vi "myRIO_BRig_FPGA_v3,0__PortC.vi"() -> ()   [LabVIEW 2014]
uses:
  <vilib>/rvi/FXPMathLib/FxpDiv/subVIs/nifxpmath_Div_SimConfig.ctl
  <vilib>/rvi/FXPMathLib/FxpSinAndCos/subVIs/nifxpmath_SinAndCos_SimConfig.ctl
  <vilib>/rvi/FXPMathLib/FxpDiv/simVIs/DllFxpDivTemp_sub.vi
  <vilib>/rvi/FXPMathLib/FxpSinAndCos/simVIs/DllFxpSinAndCosTemp_sub.vi
  <vilib>/rvi/Emulation/niFpgaGetClockAttributes.vi
  <vilib>/rvi/Emulation/niFpgaSctlEmulationGetInTimedLoop.vi
  <vilib>/rvi/Emulation/niFpgaEmulationReportErrorSimple.vi
  <vilib>/rvi/eio/common/nirviEmuTemplateMethod_errors.vi
  <vilib>/rvi/Emulation/niFpgaCriticalErrorInLSC.vi
  <vilib>/rvi/FXPMathLib/FxpDiv/XNode/nifxpmath_Div.xnode
  <vilib>/rvi/FXPMathLib/FxpMul/XNode/nifxpmath_Multiplier.xnode
  <vilib>/rvi/FXPMathLib/FxpSinAndCos/XNode/nifxpmath_SinAndCos.xnode
  <vilib>/rvi/FXPMathLib/FxpSub/XNode/nifxpmath_Sub.xnode
  <vilib>/eio/EIONode/EIONode.xnode
  <vilib>/rvi/FXPMathLib/sim/FxpSim.dll
panel:
  in  "f_time_select":u32=173
  in  "laser_Nvalley":u32=100
  in  "laser_Npeak":u32=100
  in  "laserledMTrig":bool
  in  "tCycle_laser_wro":u32=100
  in  "tDelay_laser_wro":u32
  in  "tCycle_laser_rew":u32=100
  in  "tDelay_laser_rew":u32
  in  "laserResponse_reward_LED":bool
  in  "laserResponse_wrong_LED":bool
  out "SelectWrong":bool
  out "SelectReward":bool
  in  "laserResponse_wrong":bool
  in  "laserResponse_reward":bool
  in  "Left(F)_or_Right(T)":bool
  in  "ignoreWrong":bool
  in  "SelectionState":bool
  in  "laserMTrig":bool
  in  "FPGA_Stop":bool
  in  "audioTrigger_L":bool
  in  "audioTrigger_R":bool
  in  "audioFreq_L_Hz":u16=1000 min=1000 max=14000 step=1000
  in  "audioAmp_L":u16=1 min=1 max=32767 step=1
  in  "audioFreq_R_Hz":u16=1000 min=1000 max=14000 step=1000
  in  "audioAmp_R":u16=1 min=1 max=32767 step=1
  in  "A3_SL":bool
  in  "A1_SR":bool
  in  "Counts_Reset":bool
  out "A4_LickR":u32
  out "A2_LickL":u32
  in  "A6_Act":bool
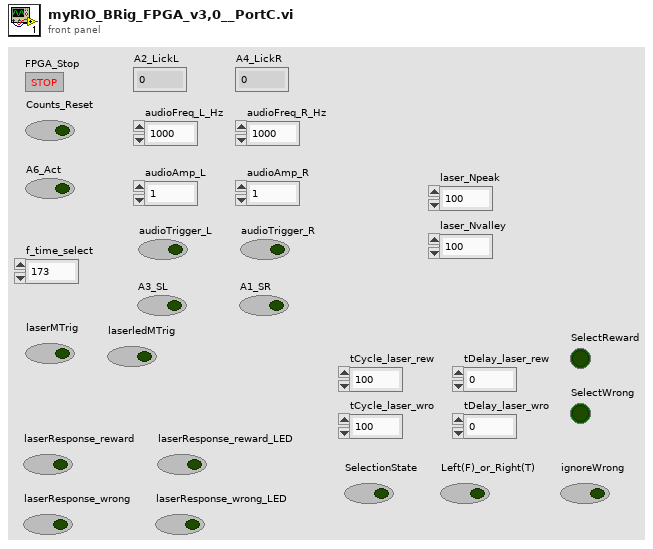
[diagram p1: front panel]
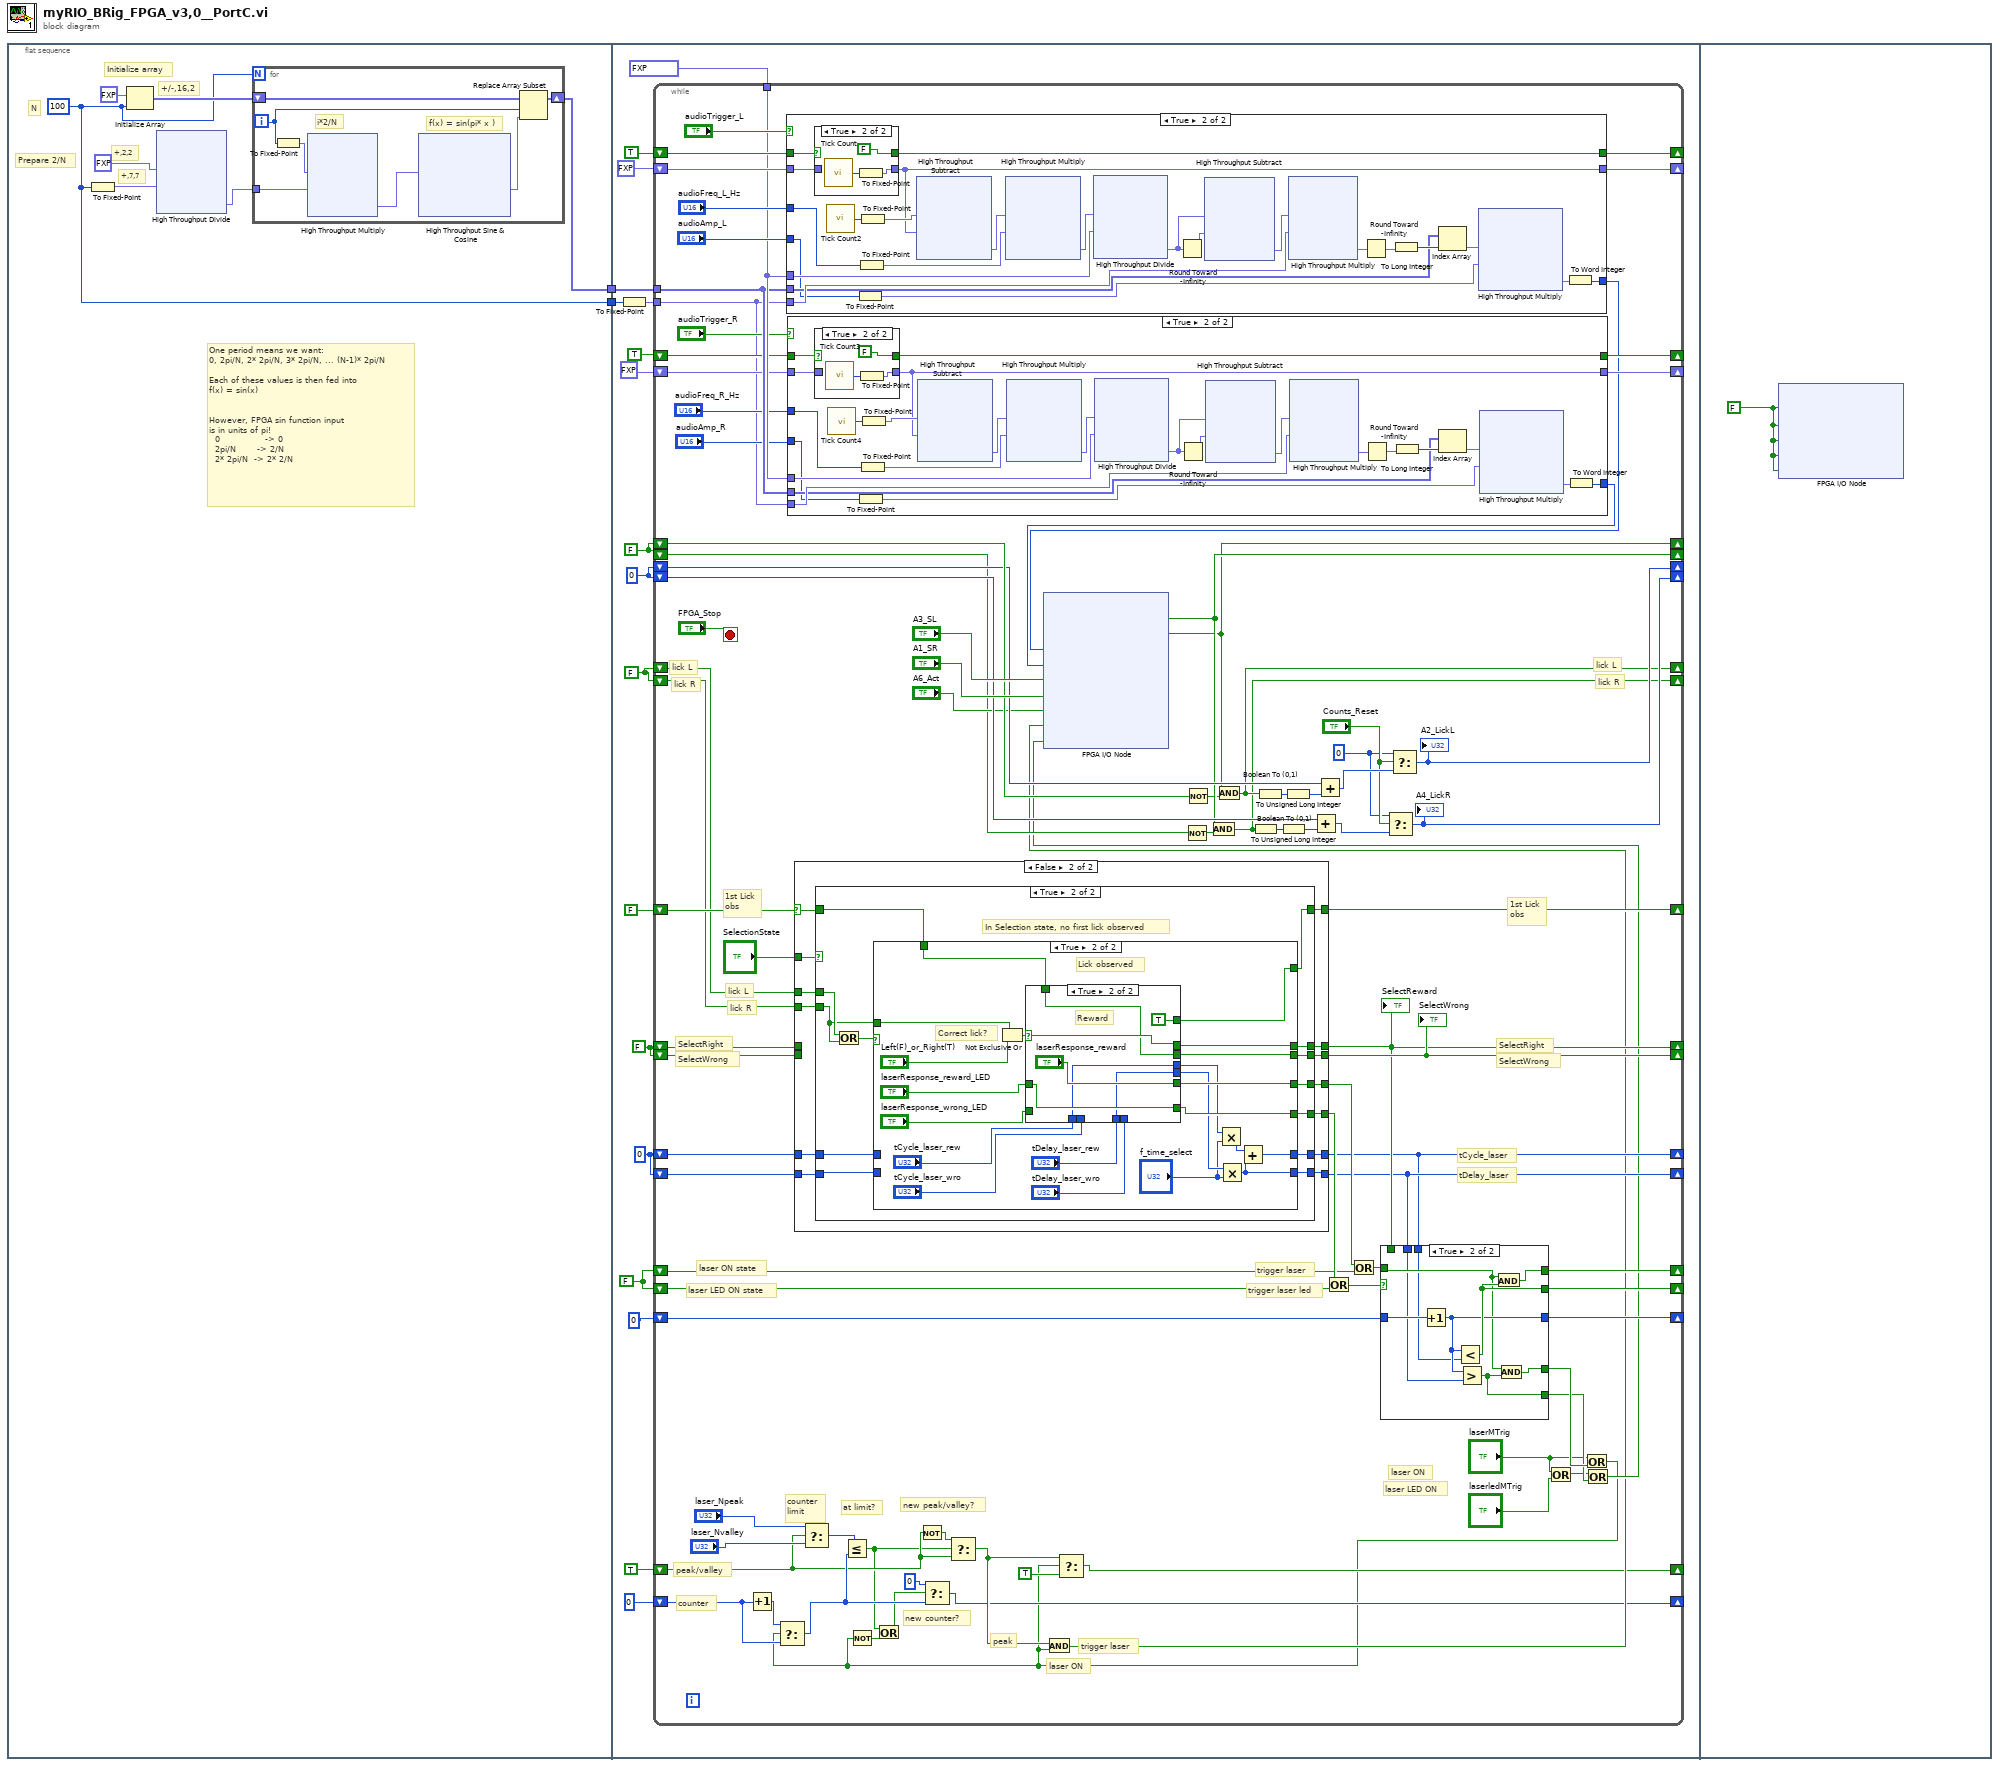
[diagram p0: block diagram]
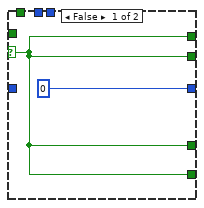
[diagram p2: hidden frame]
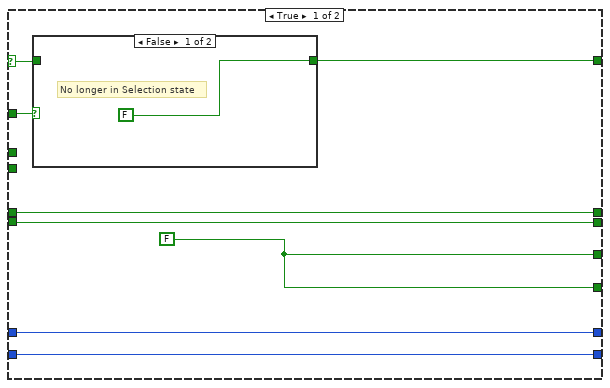
[diagram p3: hidden frame]
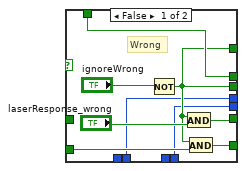
[diagram p7: hidden frame]
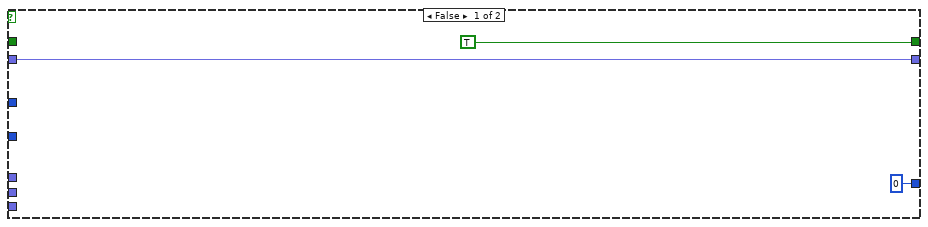
[diagram p8: hidden frame]
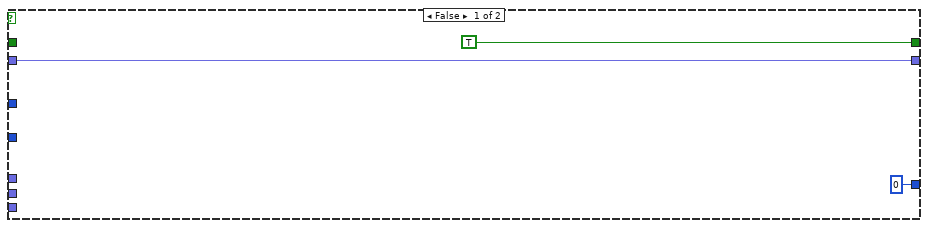
[diagram p10: hidden frame]
diagram:
  n1 = flat-sequence {
    tunnel: [w4] -> w2
    tunnel: [w3] -> w1
    tunnel: w2 -> [w86]
    tunnel: w1 -> [w88]
    frame #0 {
      w3 = 100 ("dimension size")
      # "N"
      # "+,7,7"
      # "+,2,2"
      # "+/-,16,2"
      # "Prepare 2/N"
      # "One period means we want:\n0, 2pi/N, 2* 2pi/N, 3* 2pi/N, ... (N-1)* 2pi/N\n\nEach of these values is then fed into\nf(x) = sin(x)\n\n\nHowever, FPGA sin function input\nis in units of pi!\n  0               -> 0\n  2pi/N       -> 2/N\n  2* 2pi/N  -> 2* 2/N"
      # "Initialize array"
      n2 = To Fixed-Point(number=w3) -> (fixed-point=w6:fxp<+,7,7>)  [unwired: 1 in]
      n3 = Initialize Array(fxp<+/-,16,2> 0.0 ("element"), w3) -> (w9:fxp<+/-,16,2>[])
      n4 = xnode "High Throughput Divide"("x"=fxp<+,2,2> 2.0, "y"=w6) -> ("x/y"=w5:fxp<+,27,0>)
      n5 = for {
        N: w3 -> [_]
        shift-right: [w42] -> w4
        shift-left: w9 -> [w43]
        tunnel: w5 -> [w38]
        i -> [w41]
        # "f(x) = sin(pi* x )"
        # "i*2/N"
        n6 = To Fixed-Point(number=w41) -> (fixed-point=w39:fxp<+,7,7>)  [unwired: 1 in]
        n7 = xnode ("High Throughput Multiply")("x"=w39, "y"=w38) -> ("x*y"=w37:fxp<+,34,7>)
        n8 = xnode "High Throughput Sine & Cosine"("x (pi)"=w37) -> ("sin(x)"=w40:fxp<+/-,16,2>)  [unwired: 1 out]
        n9 = Replace Array Subset(array=w43, new element=w40, index=w41) -> (w42:fxp<+/-,16,2>[])
      }
    }
    frame #1 {
      w76 = u32 0
      w78 = FALSE
      w77 = FALSE
      w81 = FALSE
      w82 = FALSE
      w83 = u32 0
      n10 = To Fixed-Point(number=w88) -> (fixed-point=w87:fxp<+,7,7>)  [unwired: 1 in]
      n11 = while {
        shift-right: [w175] -> _
        shift-left: TRUE -> [w179]
        shift-right: [w174] -> _
        shift-left: fxp<+,32,32> 0.0 -> [w178]
        tunnel: fxp<+,17,26> 40000000.0 -> [w173]
        tunnel: w87 -> [w166]
        tunnel: w86 -> [w172]
        shift-right: [w165] -> _
        shift-left: TRUE -> [w171]
        shift-right: [w164] -> _
        shift-left: fxp<+,32,32> 0.0 -> [w170]
        shift-right: [w141] -> _
        shift-left: w83 -> [w153]
        shift-right: [w144] -> _
        shift-left: w83 -> [w157]
        shift-right: [w145] -> _
        shift-left: w82 -> [w148]
        shift-right: [w142] -> _
        shift-left: w82 -> [w154]
        shift-right: [w139] -> _
        shift-left: FALSE -> [w138]
        shift-right: [w137] -> _
        shift-left: w81 -> [w135]
        shift-right: [w136] -> _
        shift-left: w81 -> [w134]
        shift-right: [w124] -> _
        shift-left: w77 -> [w126]
        shift-right: [w132] -> _
        shift-left: u32 0 -> [w133]
        shift-right: [w118] -> _
        shift-left: w78 -> [w130]
        shift-right: [w131] -> _
        shift-left: w78 -> [w129]
        shift-right: [w125] -> _
        shift-left: w77 -> [w122]
        shift-right: [w114] -> _
        shift-left: w76 -> [w117]
        shift-right: [w115] -> _
        shift-left: w76 -> [w116]
        shift-right: [w96] -> _
        shift-left: u32 0 -> [w108]
        shift-right: [w97] -> _
        shift-left: TRUE -> [w100]
        stop <- "FPGA_Stop" stop-if-true
        w150 = u32 0
        # "trigger laser"
        # "peak"
        # "laser ON"
        # "new peak/valley?"
        # "counter"
        # "peak/valley"
        # "new counter?"
        # "at limit?"
        # "counter\nlimit"
        # "tDelay_laser"
        # "tCycle_laser"
        # "laser LED ON"
        # "laser ON"
        # "laser LED ON state"
        # "laser ON state"
        # "SelectWrong"
        # "SelectRight"
        # "SelectWrong"
        # "SelectRight"
        # "lick R"
        # "lick L"
        # "1st Lick\nobs"
        # "1st Lick\nobs"
        # "lick R"
        # "lick L"
        # "lick R"
        # "lick L"
        # "trigger laser led"
        # "trigger laser"
        n12 = Increment(x=w108) -> (x+1=w106:u32)
        n13 = case shown="True" "audioTrigger_L" {
          tunnel: w179 -> [_ w357]
          tunnel: w178 -> [w333 w356]
          tunnel: "audioFreq_L_Hz" -> [_ w353]
          tunnel: w173 -> [_ w350]
          tunnel: [w333 w334] -> w174
          tunnel: [TRUE w347] -> w175
          tunnel: w166 -> [_ w346]
          tunnel: w172 -> [_ w341]
          tunnel: "audioAmp_L" -> [_ w339]
          tunnel: [i16 0 w336] -> w160
          frame False {
          }
          frame True {
            n14 = case shown="True" w357 {
              selector: w357 -> [w386 _]
              tunnel: [w386 FALSE] -> w347
              tunnel: w356 -> [w385 _]
              tunnel: [w385 w387] -> w334
              frame False {
              }
              frame True {
                n15 = call "Tick Count"() -> ("Tick Count(Ticks)"=w389:u32)
                n16 = To Fixed-Point(number=w389) -> (fixed-point=w387:fxp<+,32,32>)  [unwired: 1 in]
              }
            }
            n17 = call "Tick Count2"() -> ("Tick Count(Ticks)"=w355:u32)
            n18 = To Fixed-Point(number=w339) -> (fixed-point=w338:fxp<+,15,15>)  [unwired: 1 in]
            n19 = To Fixed-Point(number=w353) -> (fixed-point=w352:fxp<+,14,14>)  [unwired: 1 in]
            n20 = To Fixed-Point(number=w355) -> (fixed-point=w335:fxp<+,32,32>)  [unwired: 1 in]
            n21 = xnode "High Throughput Subtract"("x"=w335, "y"=w334) -> ("x-y"=w354:fxp<+,32,32>)
            n22 = xnode ("High Throughput Multiply")("x"=w354, "y"=w352) -> ("x*y"=w351:fxp<+,46,46>)
            n23 = xnode "High Throughput Divide"("x"=w351, "y"=w350) -> ("x/y"=w349:fxp<+,34,21>)
            n24 = Round Toward -Infinity(1:w349) -> (0:w348:fxp<+,21,21>)
            n25 = xnode "High Throughput Subtract"("x"=w349, "y"=w348) -> ("x-y"=w345:fxp<+,14,1>)
            n26 = xnode ("High Throughput Multiply")("x"=w345, "y"=w346) -> ("x*y"=w342:fxp<+,21,8>)
            n27 = Round Toward -Infinity(1:w342) -> (0:w344:fxp<+,8,8>)
            n28 = To Long Integer(number=w344) -> (32bit integer=w343:i32)
            n29 = Index Array(array=w341, index=w343) -> (element=w340:fxp<+/-,16,2>)
            n30 = xnode ("High Throughput Multiply")("x"=w340, "y"=w338) -> ("x*y"=w337:fxp<+/-,31,17>)
            n31 = To Word Integer(number=w337) -> (16bit integer=w336:i16)
          }
        }
        n32 = case shown="True" "audioTrigger_R" {
          tunnel: w171 -> [_ w298]
          tunnel: w170 -> [w274 w297]
          tunnel: "audioFreq_R_Hz" -> [_ w294]
          tunnel: w173 -> [_ w291]
          tunnel: [w274 w275] -> w164
          tunnel: [TRUE w288] -> w165
          tunnel: w166 -> [_ w287]
          tunnel: w172 -> [_ w282]
          tunnel: "audioAmp_R" -> [_ w280]
          tunnel: [i16 0 w277] -> w161
          frame False {
          }
          frame True {
            n33 = case shown="True" w298 {
              selector: w298 -> [w327 _]
              tunnel: [w327 FALSE] -> w288
              tunnel: w297 -> [w326 _]
              tunnel: [w326 w328] -> w275
              frame False {
              }
              frame True {
                n34 = call "Tick Count3"() -> ("Tick Count(Ticks)"=w330:u32)
                n35 = To Fixed-Point(number=w330) -> (fixed-point=w328:fxp<+,32,32>)  [unwired: 1 in]
              }
            }
            n36 = call "Tick Count4"() -> ("Tick Count(Ticks)"=w296:u32)
            n37 = To Fixed-Point(number=w280) -> (fixed-point=w279:fxp<+,15,15>)  [unwired: 1 in]
            n38 = To Fixed-Point(number=w294) -> (fixed-point=w293:fxp<+,14,14>)  [unwired: 1 in]
            n39 = To Fixed-Point(number=w296) -> (fixed-point=w276:fxp<+,32,32>)  [unwired: 1 in]
            n40 = xnode "High Throughput Subtract"("x"=w276, "y"=w275) -> ("x-y"=w295:fxp<+,32,32>)
            n41 = xnode ("High Throughput Multiply")("x"=w295, "y"=w293) -> ("x*y"=w292:fxp<+,46,46>)
            n42 = xnode "High Throughput Divide"("x"=w292, "y"=w291) -> ("x/y"=w290:fxp<+,34,21>)
            n43 = Round Toward -Infinity(1:w290) -> (0:w289:fxp<+,21,21>)
            n44 = xnode "High Throughput Subtract"("x"=w290, "y"=w289) -> ("x-y"=w286:fxp<+,14,1>)
            n45 = xnode ("High Throughput Multiply")("x"=w286, "y"=w287) -> ("x*y"=w283:fxp<+,21,8>)
            n46 = Round Toward -Infinity(1:w283) -> (0:w285:fxp<+,8,8>)
            n47 = To Long Integer(number=w285) -> (32bit integer=w284:i32)
            n48 = Index Array(array=w282, index=w284) -> (element=w281:fxp<+/-,16,2>)
            n49 = xnode ("High Throughput Multiply")("x"=w281, "y"=w279) -> ("x*y"=w278:fxp<+/-,31,17>)
            n50 = To Word Integer(number=w278) -> (16bit integer=w277:i16)
          }
        }
        n51 = case shown="False" w138 {
          selector: w138 -> [w198 w213]
          tunnel: "SelectionState" -> [w200 w215]
          tunnel: [w199 w214] -> w139
          tunnel: w135 -> [_ w212]
          tunnel: w134 -> [_ w211]
          tunnel: [w197 w210] -> w123
          tunnel: [w195 w209] -> w118
          tunnel: [w196 w208] -> w131
          tunnel: w130 -> [w195 _]
          tunnel: w129 -> [w196 _]
          tunnel: [w197 w207] -> w127
          tunnel: [w194 w206] -> w114
          tunnel: [w193 w205] -> w115
          tunnel: w117 -> [w194 w204]
          tunnel: w116 -> [w193 w203]
          frame True {
            w197 = FALSE
            n52 = case shown="False" w200 {
              tunnel: [FALSE w202] -> w199
              tunnel: w198 -> [_ w202]
              frame False {
                # "No longer in Selection state"
              }
              frame True {
                # "Already observed first lick, no other action"
              }
            }
          }
          frame False {
            n53 = case shown="True" w215 {
              tunnel: [w218 w228] -> w214
              tunnel: w213 -> [w218 w224]
              tunnel: w212 -> [_ w230]
              tunnel: w211 -> [_ w229]
              tunnel: [w218 w227] -> w210
              tunnel: [w218 w226] -> w209
              tunnel: [w218 w225] -> w208
              tunnel: [w218 w223] -> w207
              tunnel: [w217 w222] -> w206
              tunnel: [w216 w221] -> w205
              tunnel: w204 -> [w217 w220]
              tunnel: w203 -> [w216 w219]
              frame False {
                # "Not in Selection state"
              }
              frame True {
                # "In Selection state, no first lick observed"
                n54 = Or(x=w230, y=w229) -> (x .or. y?=w231:bool)
                n55 = case shown="True" w231 {
                  tunnel: w229 -> [_ w254]
                  tunnel: [w234 w247] -> w228
                  tunnel: [w234 w252] -> w227
                  tunnel: [w234 w251] -> w226
                  tunnel: [w234 w250] -> w225
                  tunnel: w224 -> [w234 w249]
                  tunnel: [w234 w248] -> w223
                  tunnel: [w233 w236] -> w222
                  tunnel: [w232 w235] -> w221
                  tunnel: w220 -> [w233 _]
                  tunnel: w219 -> [w232 _]
                  frame False {
                  }
                  frame True {
                    # "Correct lick?"
                    # "Lick observed"
                    n56 = Not Exclusive Or(1:"Left(F)_or_Right(T)", 2:w254) -> (0:w253:bool)
                    n57 = case shown="True" w253 {
                      selector: w253 -> [_ w270]
                      tunnel: [w261 "laserResponse_reward"] -> w252
                      tunnel: [w259 w266] -> w250
                      tunnel: [w263 w270] -> w251
                      tunnel: w249 -> [w263 w266]
                      tunnel: [w260 w268] -> w248
                      tunnel: [w259 TRUE] -> w247
                      tunnel: "laserResponse_reward_LED" -> [_ w268]
                      tunnel: "laserResponse_wrong_LED" -> [w258 _]
                      tunnel: "tCycle_laser_rew" -> [_ w265]
                      tunnel: "tCycle_laser_wro" -> [w256 _]
                      tunnel: "tDelay_laser_rew" -> [_ w267]
                      tunnel: "tDelay_laser_wro" -> [w257 _]
                      tunnel: [w257 w267] -> w239
                      tunnel: [w256 w265] -> w238
                      frame False {
                        # "Wrong"
                        n58 = Not(x="ignoreWrong") -> (.not. x?=w259:bool)
                        n59 = And(x=w259, y="laserResponse_wrong") -> (x .and. y?=w261:bool)
                        n60 = And(x=w259, y=w258) -> (x .and. y?=w260:bool)
                      }
                      frame True {
                        # "Reward"
                      }
                    }
                    n61 = Multiply(x=w238, y="f_time_select") -> (x*y=w240:u32)
                    n62 = Multiply(x=w239, y="f_time_select") -> (x*y=w235:u32)
                    n63 = Add(x=w240, y=w235) -> (x+y=w236:u32)
                  }
                }
              }
            }
          }
        }
        "SelectWrong" <- w131
        "SelectReward" <- w118
        n64 = Select(t="laser_Npeak", s=w100, f="laser_Nvalley") -> (s? t:f=w110:u32)
        n65 = Not(x=w100) -> (.not. x?=w101:bool)
        n66 = Not(x=w148) -> (.not. x?=w147:bool)
        n67 = Not(x=w154) -> (.not. x?=w143:bool)
        n68 = Or(x=w127, y=w126) -> (x .or. y?=w128:bool)
        n69 = Or(x=w123, y=w122) -> (x .or. y?=w121:bool)
        n70 = case shown="True" w128 {
          selector: w128 -> [w182 _]
          tunnel: w133 -> [_ w192]
          tunnel: [u32 0 w189] -> w132
          tunnel: [w182 w190] -> w124
          tunnel: [w182 w191] -> w125
          tunnel: w121 -> [_ w188]
          tunnel: [w182 w187] -> w119
          tunnel: [w182 w186] -> w120
          tunnel: w118 -> [_ _]
          tunnel: w115 -> [_ w185]
          tunnel: w114 -> [_ w184]
          frame False {
          }
          frame True {
            n71 = Increment(x=w192) -> (x+1=w189:u32)
            n72 = Less?(x=w189, y=w184) -> (x < y?=w190:bool)
            n73 = Greater?(x=w189, y=w185) -> (0:w187:bool)
            n74 = And(x=w188, y=w190) -> (x .and. y?=w191:bool)
            n75 = And(x=w188, y=w187) -> (x .and. y?=w186:bool)
          }
        }
        n76 = Or(x="laserMTrig", y="laserledMTrig") -> (x .or. y?=w112:bool)
        n77 = Or(x="laserMTrig", y=w120) -> (x .or. y?=w94:bool)
        n78 = Select(t=w106, s=w94, f=w108) -> (s? t:f=w105:u32)
        n79 = Less Or Equal?(x=w110, y=w105) -> (x <= y?=w93:bool)
        n80 = Not(x=w94) -> (.not. x?=w95:bool)
        n81 = Or(x=w93, y=w95) -> (x .or. y?=w92:bool)
        n82 = Select(t=u32 0, s=w92, f=w105) -> (s? t:f=w96:u32)
        n83 = Select(t=w101, s=w93, f=w100) -> (s? t:f=w99:bool)
        n84 = And(x=w99, y=w94) -> (x .and. y?=w102:bool)
        n85 = Select(t=w99, s=w94, f=TRUE) -> (s? t:f=w97:bool)
        n86 = Or(x=w112, y=w119) -> (x .or. y?=w107:bool)
        n87 = xnode "FPGA I/O Node"("AudioOut/Left"=w160, "AudioOut/Right"=w161, "ConnectorC/DIO3"="A3_SL", "ConnectorC/DIO1"="A1_SR", "ConnectorC/DIO6"="A6_Act", "ConnectorC/DIO0"=w102, "ConnectorC/DIO7"=w107) -> ("ConnectorC/DIO4"=w145:bool, "ConnectorC/DIO2"=w142:bool)  [unwired: 9 in, 9 out]
        n88 = And(x=w145, y=w147) -> (x .and. y?=w136:bool)
        n89 = And(x=w142, y=w143) -> (x .and. y?=w137:bool)
        n90 = Boolean To (0,1)(Boolean=w136) -> (0, 1=w159:i16)
        n91 = Boolean To (0,1)(Boolean=w137) -> (0, 1=w156:i16)
        n92 = To Unsigned Long Integer(number=w159) -> (unsigned 32bit integer=w158:u32)
        n93 = To Unsigned Long Integer(number=w156) -> (unsigned 32bit integer=w155:u32)
        n94 = Add(x=w157, y=w158) -> (x+y=w146:u32)
        n95 = Add(x=w153, y=w155) -> (x+y=w152:u32)
        n96 = Select(t=w150, s="Counts_Reset", f=w146) -> (s? t:f=w144:u32)
        "A4_LickR" <- w144
        n97 = Select(t=w150, s="Counts_Reset", f=w152) -> (s? t:f=w141:u32)
        "A2_LickL" <- w141
      }
    }
    frame #2 {
      w390 = FALSE ("ConnectorA/DIO3")
      n98 = xnode "FPGA I/O Node"("ConnectorC/DIO3"=w390, "ConnectorC/DIO1"=w390, "ConnectorC/DIO0"=w390, "ConnectorC/DIO6"=w390, "ConnectorC/DIO7"=w390) -> ()  [unwired: 5 in, 5 out]
    }
  }
